vi "GarbageCollector.vi"(1 "full class name":string, 3 "only from same owner as caller? (T)":bool=TRUE, 5 "error in (no error)":errorcluster) -> (14 "OK":bool, 15 "# of objects killed":i32, 19 "error out":errorcluster)   [LabVIEW 2020, in "G#Object.lvclass"]
doc: "If 'full class name' is empty string, garbage collector will execute the Destroy method on all remaining objects. It will also clear and close all remaining queues, data value and event references and make sure there are no memory leaks.\n\nUse this VI as the last of all VIs in your program. It will make sure that your application exits without any leaks."
uses:
  <vilib>/addons/_AddQ/G#Object/G#Object.lvclass
  <vilib>/addons/_AddQ/G#Object/utils/G#Object_EventType.ctl
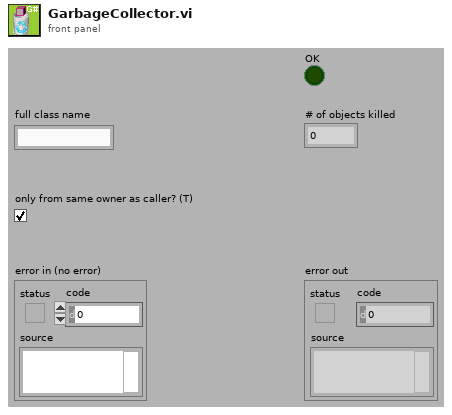
[diagram p1: front panel]
types:
  T1 = typedef "G#Object.lvclass/G#Object_EventType.ctl" = enum16{"Created new", "Looked up existing", "Deleted", "Forced delete", "Not deleted", "Garbage collected", "Cleared", "User", "Error", "External create object", "External create class attributes", "Created class attributes", "Run constructor", "Run constructor done", "Run open method", "Run open method done"}
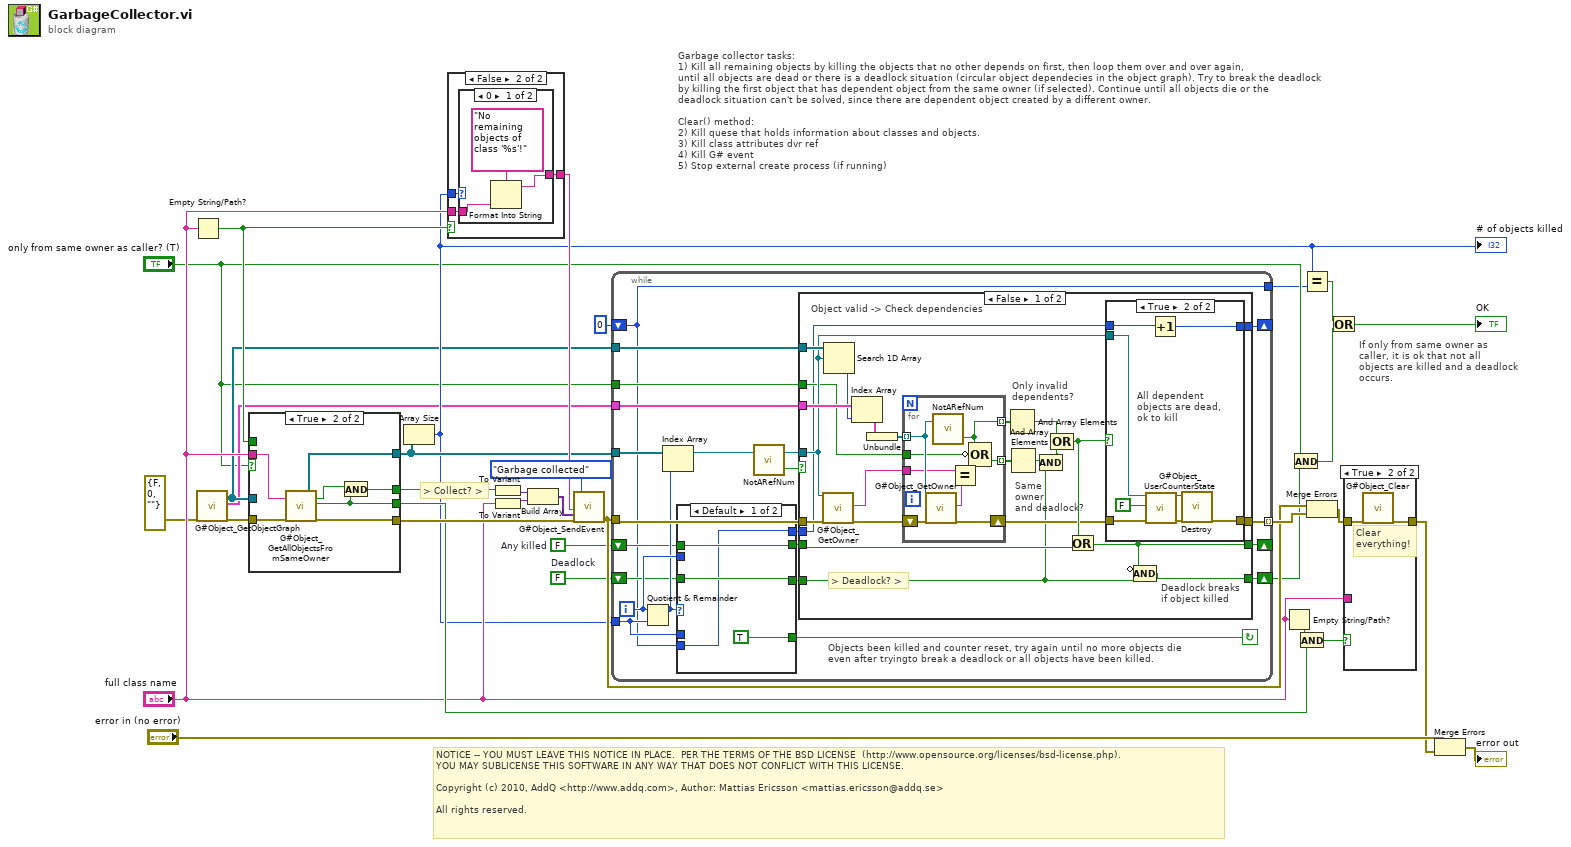
[diagram p0: block diagram]
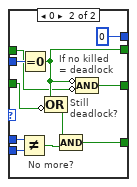
[diagram p2: hidden frame]
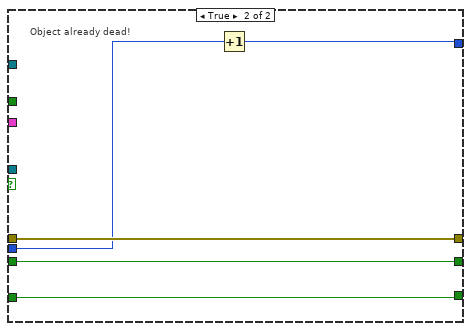
[diagram p4: hidden frame]
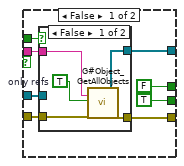
[diagram p5: hidden frame]
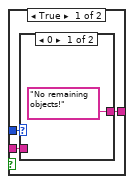
[diagram p7: hidden frame]
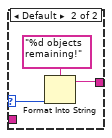
[diagram p8: hidden frame]
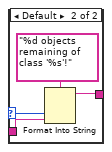
[diagram p9: hidden frame]
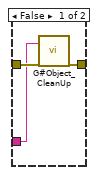
[diagram p10: hidden frame]
diagram:
  w8 = FALSE  # Deadlock
  w12 = FALSE  # Any killed
  # "If only from same owner as\ncaller, it is ok that not all\nobjects are killed and a deadlock\noccurs."
  # "> Collect? >"
  # "Garbage collector tasks:\n1) Kill all remaining objects by killing the objects that no other depends on first, then loop them over and over again,\nuntil all objects are dead or there is a deadlock situation (circular object dependecies in the object graph). Try to break the deadlock\nby killing the first object that has dependent object from the same owner (if selected). Continue until all objects die or the\ndeadlock situation can't be solved, since there are dependent object created by a different owner.\n\nClear() method:\n2) Kill quese that holds information about classes and objects.\n3) Kill class attributes dvr ref\n4) Kill G# event\n5) Stop external create process (if running)"
  # "NOTICE -- YOU MUST LEAVE THIS NOTICE IN PLACE.  PER THE TERMS OF THE BSD LICENSE  (http://www.opensource.org/licenses/bsd-license.php).\nYOU MAY SUBLICENSE THIS SOFTWARE IN ANY WAY THAT DOES NOT CONFLICT WITH THIS LICENSE.\n\nCopyright (c) 2010, AddQ <http://www.addq.com>, Author: Mattias Ericsson <mattias.ericsson@addq.se>\n\nAll rights reserved."
  n1 = Empty String/Path?(string/path="full class name") -> (empty?=w15:bool)
  n2 = call <vilib>:"G#Object_GetObjectGraph.vi"("error in (no error)"=errorcluster {"status"=FALSE, "code"=0, "source"=""}) -> ("all refs"=w7:refnum<class "G#Object.lvclass">[], "dependent objects"=w6:cluster{refnum<class "G#Object.lvclass">[]}[], "error out"=w13:errorcluster)  [unwired: 16 in]
  n3 = case shown="True" "only from same owner as caller? (T)" {
    tunnel: w13 -> [w41 w55]
    tunnel: [w40 w54] -> w28
    tunnel: [w39 w52] -> w27
    tunnel: "full class name" -> [w38 w53]
    tunnel: [TRUE ("No other owners") w50] -> w21
    tunnel: [FALSE w49] -> w16
    tunnel: w15 -> [w35 _]
    tunnel: w7 -> [w34 _]
    frame False {
      n4 = case shown="False" w35 {
        tunnel: w41 -> [w46 w48]
        tunnel: [w45 w48] -> w40
        tunnel: [w44 w47] -> w39
        tunnel: w38 -> [w42 _]
        tunnel: w34 -> [_ w47]
        frame False {
          w43 = TRUE  # only refs
          n5 = call <vilib>:"G#Object_GetAllObjects.vi"("full class name (\"\")"=w42, "only refs (F)"=w43, "error in (no error)"=w46) -> ("all refs"=w44:refnum<class "G#Object.lvclass">[], "error out"=w45:errorcluster)  [unwired: 13 in, 2 out]
        }
        frame True {
        }
      }
    }
    frame True {
      n6 = call <vilib>:"G#Object_GetAllObjectsFromSameOwner.vi"("full class name (\"\")"=w53, "error in (no error)"=w55) -> ("all refs"=w52:refnum<class "G#Object.lvclass">[], "external creator process owns"=w51:bool, "no other owners"=w50:bool, "error out"=w54:errorcluster)  [unwired: 14 in]
      n7 = And(x=w51, y=w50) -> (x .and. y?=w49:bool)
    }
  }
  n8 = Array Size(array=w27) -> (size(s)=w10:i32)
  "# of objects killed" <- w10
  n9 = case shown="False" w15 {
    tunnel: [w58 w65] -> w29
    tunnel: w10 -> [w57 w64]
    tunnel: "full class name" -> [w56 w63]
    frame True {
      n10 = case shown="0" w57 {
        selector: w57 -> [_ w61]
        tunnel: ["No remaining objects!" w60] -> w58
        tunnel: w56 -> [_ _]
        frame 0 {
        }
        frame Default {
          n11 = Format Into String(format string="%d objects remaining!", w61) -> (resulting string=w60:string)  [unwired: 2 in, 1 out]
        }
      }
    }
    frame False {
      n12 = case shown="0" w64 {
        selector: w64 -> [_ w71]
        tunnel: [w67 w70] -> w65
        tunnel: w63 -> [w66 w69]
        frame 0 {
          n13 = Format Into String(format string="No remaining objects of class '%s'!", w66) -> (resulting string=w67:string)  [unwired: 2 in, 1 out]
        }
        frame Default {
          n14 = Format Into String(format string="%d objects remaining of class '%s'!", w71, w69) -> (resulting string=w70:string)  [unwired: 2 in, 1 out]
        }
      }
    }
  }
  n15 = To Variant(anything=w16) -> (Variant=w20:variant)
  n16 = To Variant(anything="full class name") -> (Variant=w19:variant)
  n17 = Build Array(w20, w19) -> (w18:variant[])
  n18 = call <vilib>:"G#Object_SendEvent.vi"("comment"=w29, "parameters"=w18, "error in (no error)"=w28, "G# event type"=G#Object_EventType."Garbage collected" ("G#Event")) -> ("error out"=w24:errorcluster)  [unwired: 15 in]
  n19 = while {
    tunnel: w24 -> [w94]
    tunnel: [w92] -> w33 mode=indexing
    tunnel: w7 -> [w90]
    tunnel: w6 -> [w87]
    shift-right: [w86] -> _
    shift-left: w12 -> [w82]
    tunnel: w27 -> [w91]
    tunnel: w10 -> [w79]
    shift-right: [w80] -> _
    shift-left: 0 -> [w73]
    tunnel: "only from same owner as caller? (T)" -> [w78]
    shift-right: [w75] -> w2
    shift-left: w8 -> [w77]
    tunnel: [w73] -> w1
    i -> [w85]
    stop <- w81 continue-if-true
    # "Objects been killed and counter reset, try again until no more objects die\neven after tryingto break a deadlock or all objects have been killed."
    n20 = Quotient & Remainder(x=w85, y=w79) -> (x-y*floor(x/y)=w84:i32)  [unwired: 1 out]
    n21 = Index Array(array=w91, index=w84) -> (element=w89:refnum<class "G#Object.lvclass">)
    n22 = case shown="Default" w84 {
      tunnel: w85 -> [_ w109]
      tunnel: [w98 w105] -> w83
      tunnel: w82 -> [w98 w104]
      tunnel: [TRUE w108] -> w81
      tunnel: w79 -> [_ w102]
      tunnel: w77 -> [w96 w107]
      tunnel: [w96 w103] -> w76
      tunnel: w73 -> [w95 w101]
      tunnel: [w95 0] -> w74
      frame Default {
      }
      frame 0 {
        # "If no killed\n= deadlock"
        # "Still\ndeadlock?"
        # "No more?"
        n23 = Not Equal?(x=w102, y=w101) -> (x != y?=w100:bool)
        n24 = Equal To 0?(x=w109) -> (x = 0?=w105:bool)
        n25 = Compound Arithmetic op=OR(w105, invert w107) -> (w106:bool)
        n26 = Compound Arithmetic op=AND(w106, w100) -> (w108:bool)
        n27 = Compound Arithmetic op=AND(invert w105, invert w104) -> (w103:bool)
      }
    }
    n28 = call-dynamic "NotARefNum.vi"("reference in"=w89) -> ("not a refnum?"=w88:bool, "reference out"=w93:refnum<class "G#Object.lvclass">)  [unwired: 1 in]
    n29 = case shown="False" w88 {
      tunnel: w94 -> [w126 w157]
      tunnel: w93 -> [w125 _]
      tunnel: [w133 w157] -> w92
      tunnel: w90 -> [w132 _]
      tunnel: w87 -> [w131 _]
      tunnel: w83 -> [w129 w156]
      tunnel: [w121 w156] -> w86
      tunnel: [w128 w153] -> w80
      tunnel: w78 -> [w113 _]
      tunnel: w76 -> [w119 w155]
      tunnel: [w120 w155] -> w75
      tunnel: w74 -> [w110 w154]
      frame False {
        # "Only invalid\ndependents?"
        # "Same\nowner\nand deadlock?"
        # "> Deadlock? >"
        # "Deadlock breaks\nif object killed"
        # "Object valid -> Check dependencies"
        n30 = call-dynamic "G#Object_GetOwner.vi"("reference in"=w125, "error in (no error)"=w126) -> ("owner"=w123:string, "error out"=w124:errorcluster)  [unwired: 15 in, 1 out]
        n31 = Search 1D Array(1D array=w132, element=w125) -> (index of element=w127:i32)  [unwired: 1 in]
        n32 = Index Array(array=w131, index=w127) -> (element=w118:cluster{refnum<class "G#Object.lvclass">[]})
        n33 = Unbundle(w118) -> (w117:refnum<class "G#Object.lvclass">[])
        n34 = for {
          tunnel: w117 -> [w140] mode=indexing
          tunnel: [w137] -> w116 mode=indexing
          tunnel: w123 -> [w139]
          tunnel: [w135] -> w115 mode=indexing
          tunnel: w113 -> [w134]
          shift-right: [w141] -> w122
          shift-left: w124 -> [w142]
          n35 = call-dynamic "G#Object_GetOwner.vi"("reference in"=w140, "error in (no error)"=w142) -> ("owner"=w138:string, "error out"=w141:errorcluster)  [unwired: 15 in, 1 out]
          n36 = call-dynamic "NotARefNum.vi"("reference in"=w140) -> ("not a refnum?"=w137:bool)  [unwired: 1 in, 1 out]
          n37 = Equal?(x=w139, y=w138) -> (x = y?=w136:bool)
          n38 = Compound Arithmetic op=OR(w137, invert w134, w136) -> (w135:bool)
        }
        n39 = And Array Elements(Boolean array=w116) -> (logical AND=w114:bool)
        n40 = And Array Elements(Boolean array=w115) -> (logical AND=w112:bool)
        n41 = Compound Arithmetic op=AND(w112, w119) -> (w111:bool)
        n42 = Compound Arithmetic op=OR(w114, w111) -> (w130:bool)
        n43 = Or(x=w130, y=w129) -> (x .or. y?=w121:bool)
        n44 = case shown="True" w130 {
          tunnel: w122 -> [w144 w152]
          tunnel: [w144 w149] -> w133
          tunnel: w125 -> [_ w148]
          tunnel: w110 -> [w143 w146]
          tunnel: [w143 w145] -> w128
          frame False {
            # "There are still valid\nobjects that\nis dependent of this\nobject, don't kill yet."
          }
          frame True {
            # "All dependent\nobjects are dead,\nok to kill"
            n45 = call <vilib>:"G#Object_UserCounterState.vi"("reference in"=w148, "user counter (F)"=FALSE, "error in (no error)"=w152) -> ("reference out"=w147:refnum<class "G#Object.lvclass">, "error out"=w151:errorcluster)  [unwired: 15 in]
            n46 = Increment(x=w146) -> (x+1=w145:i32)
            n47 = call-dynamic "Destroy.vi"("reference in"=w147, "error in (no error)"=w151) -> ("error out"=w149:errorcluster)  [unwired: 16 in, 1 out]
          }
        }
        n48 = Compound Arithmetic op=AND(invert w121, w119) -> (w120:bool)
      }
      frame True {
        # "Object already dead!"
        n49 = Increment(x=w154) -> (x+1=w153:i32)
      }
    }
  }
  n50 = Empty String/Path?(string/path="full class name") -> (empty?=w23:bool)
  n51 = And(x="only from same owner as caller? (T)", y=w2) -> (x .and. y?=w4:bool)
  n52 = And(x=w23, y=w21) -> (x .and. y?=w22:bool)
  n53 = Equal?(x=w10, y=w1) -> (x = y?=w3:bool)
  n54 = Merge Errors(w24, w33) -> (w26:errorcluster)
  n55 = Or(x=w3, y=w4) -> (x .or. y?=→"OK":bool)
  n56 = case shown="True" w22 {
    tunnel: w26 -> [w160 w162]
    tunnel: [w159 w161] -> w25
    tunnel: "full class name" -> [w158 _]
    frame False {
      n57 = call <vilib>:"G#Object_CleanUp.vi"("full class name (\"\")"=w158, "error in (no error)"=w160) -> ("error out"=w159:errorcluster)  [unwired: 16 in, 1 out]
    }
    frame True {
      # "Clear\neverything!"
      n58 = call <vilib>:"G#Object_Clear.vi"("error in (no error)"=w162) -> ("error out"=w161:errorcluster)  [unwired: 18 in]
    }
  }
  n59 = Merge Errors("error in (no error)", w25) -> (→"error out":errorcluster)
